vi "Main.vi"() -> ()   [LabVIEW 2013]
uses:
  <vilib>/myRIO/Instrument Drivers/Onboard IO/SPI/vis/Smart Open.vi
  <vilib>/myRIO/Instrument Drivers/Onboard IO/SPI/vis/Configure.vi
  <vilib>/myRIO/Instrument Drivers/Onboard IO/SPI/vis/Write.vi
  <vilib>/myRIO/Common/Instrument Driver Framework/myRIO v1.0/UART/vis/myRIO v1.0 Close UART.vi
  <vilib>/myRIO/Instrument Drivers/Onboard IO/SPI/vis/Open.vi
  <vilib>/myRIO/Instrument Drivers/Onboard IO/SPI/vis/Write Read.vi
  <vilib>/myRIO/Common/Instrument Driver Framework/myRIO v1.0/SPI/vis/myRIO v1.1 Open SPI.vi
  <vilib>/myRIO/Common/Instrument Driver Framework/Utilities/vis/Validate Channels.vi
  <vilib>/myRIO/Common/Instrument Driver Framework/myRIO v1.0/SPI/vis/myRIO v1.0 Reserve SPI.vi
  <vilib>/myRIO/Common/Instrument Driver Framework/myRIO v1.0/SPI/vis/myRIO v1.0 Build MUX Configuration SPI.vi
  <vilib>/myRIO/Common/Instrument Driver Framework/myRIO v1.0/Resource Manager/vis/myRIO v1.0 Reserve Channel List.vi
  <vilib>/myRIO/Common/Instrument Driver Framework/myRIO v1.0/Resource Manager/vis/myRIO v1.0 Create Configuration List.vi
  <vilib>/myRIO/Common/Instrument Driver Framework/myRIO v1.0/Resource Manager/vis/myRIO v1.0 Reserve Channel.vi
  <vilib>/myRIO/Common/Instrument Driver Framework/myRIO v1.0/Resource Manager/vis/myRIO v1.0 Unreserve Channel.vi
  <vilib>/myRIO/Common/Instrument Driver Framework/myRIO v1.0/Resource Manager/vis/myRIO v1.0 Build Mutex Name.vi
  <vilib>/myRIO/Common/Instrument Driver Framework/myRIO v1.0/myRIO v1.1 Open.vi
  <vilib>/Utility/VariantDataType/GetNumericInfo.vi
  <vilib>/Utility/error.llb/Error Cluster From Error Code.vi
  <vilib>/myRIO/Common/Instrument Driver Framework/Utilities/vis/IO Manager.vi
  <vilib>/myRIO/Common/Instrument Driver Framework/Utilities/vis/Configuration Manager.vi
  <vilib>/myRIO/Common/Instrument Driver Framework/myRIO v1.0/Resource Manager/vis/myRIO v1.0 Configure IO.vi
  <vilib>/myRIO/Common/Instrument Driver Framework/myRIO v1.0/myRIO v1.0 Close.vi
  <vilib>/myRIO/Common/Instrument Driver Framework/myRIO v1.0/SPI/vis/myRIO v1.0 Configure SPI.vi
  <vilib>/myRIO/Common/Instrument Driver Framework/myRIO v1.0/SPI/vis/myRIO v1.0 Write Read SPI.vi
  <vilib>/myRIO/Common/Instrument Driver Framework/Utilities/vis/FPGA Ref Manager.vi
  <vilib>/myRIO/Common/Instrument Driver Framework/myRIO v1.0/myRIO v1.0 Reset FPGA.vi
  <vilib>/myRIO/Instrument Drivers/Utilities/Utilities.lvlib
panel:
  out "LCD display":string
  in  "[ESC]":bool
  # "LCD (SPI) demo"
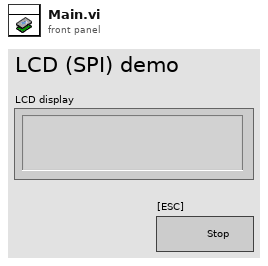
[diagram p1: front panel]
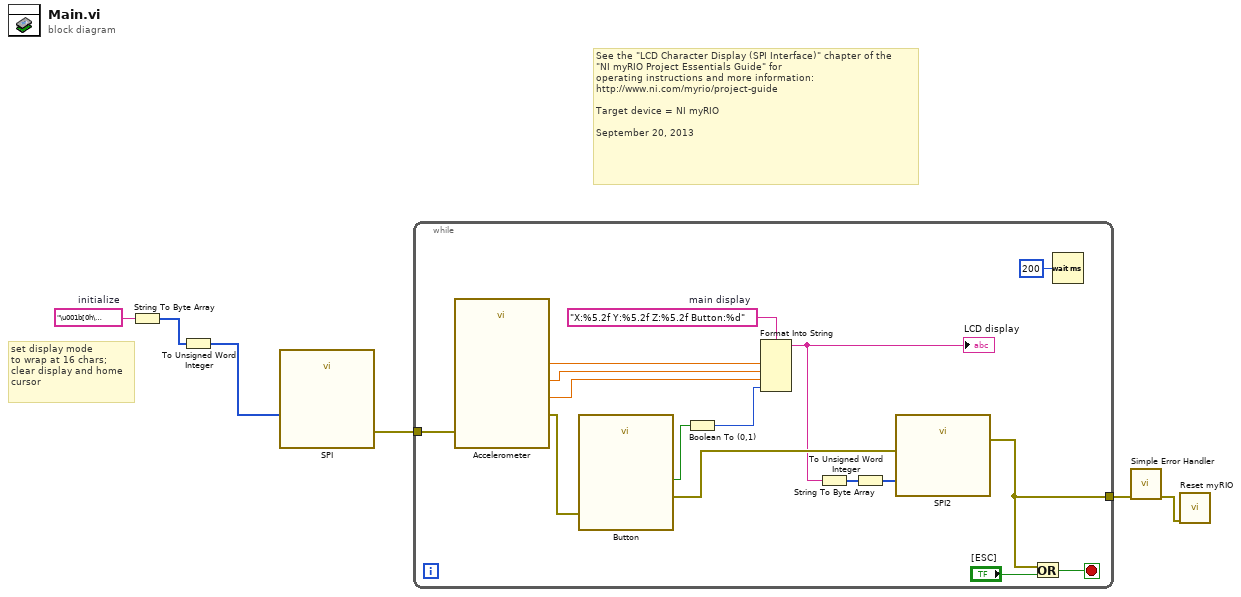
[diagram p0: block diagram]
diagram:
  w2 = "\u001b[0h\u001b[j"  # initialize
  # "See the \"LCD Character Display (SPI Interface)\" chapter of the\n\"NI myRIO Project Essentials Guide\" for\noperating instructions and more information: \nhttp://www.ni.com/myrio/project-guide\n\nTarget device = NI myRIO\n\nSeptember 20, 2013"
  # "set display mode\nto wrap at 16 chars;\nclear display and home\ncursor"
  n1 = String To Byte Array(string=w2) -> (unsigned byte array=w3:u8[])
  n2 = To Unsigned Word Integer(number=w3) -> (unsigned 16bit integer=w1:u16[])
  n3 = call "SPI"("Frames to Write"=w1) -> ("error out"=w4:errorcluster)  [unwired: 26 in]
  n4 = while {
    tunnel: [w10] -> w5
    tunnel: w4 -> [w12]
    stop <- w14 stop-if-true
    w22 = "X:%5.2f Y:%5.2f Z:%5.2f Button:%d"  # main display
    n5 = call "Accelerometer"("error in (no error)"=w12) -> ("X-Axis"=w20:dbl, "Y-Axis"=w19:dbl, "Z-Axis"=w18:dbl, "error out"=w17:errorcluster)  [unwired: 23 in]
    n6 = call "Button"("error in (no error)"=w17) -> ("Value"=w16:bool, "error out"=w11:errorcluster)  [unwired: 25 in]
    n7 = Boolean To (0,1)(Boolean=w16) -> (0, 1=w21:i16)
    n8 = Format Into String "Format Into String"(format string=w22, w20, w19, w18, w21) -> (resulting string=w8:string)  [unwired: 2 in, 1 out]
    "LCD display" <- w8
    n9 = String To Byte Array(string=w8) -> (unsigned byte array=w9:u8[])
    n10 = To Unsigned Word Integer(number=w9) -> (unsigned 16bit integer=w7:u16[])
    n11 = call "SPI2"("Frames to Write"=w7, "error in (no error)"=w11) -> ("error out"=w10:errorcluster)  [unwired: 25 in]
    n12 = Or(x=w10, y="[ESC]") -> (x .or. y?=w14:bool)
    n13 = Wait (ms)(milliseconds to wait=u32 200) -> ()  [unwired: 1 out]
  }
  n14 = call <vilib>:"Simple Error Handler.vi"("error in (no error)"=w5) -> ("error out"=w6:errorcluster)  [unwired: 4 in, 4 out]
  n15 = call <vilib>:"Reset myRIO.vi"("error in (no error)"=w6) -> ()  [unwired: 10 in, 1 out]
